vi "get_config_cluster.vi"(8 "error in (no error)":errorcluster, 11 "ScanModeDL090923Scaffold in":refnum<class "ImagingModeDL090923Scaffold.lvclass">) -> (0 "error out":errorcluster, 2 "config cluster (variant)":variant, 3 "ScanModeDL090923Scaffold out":refnum<class "ImagingModeDL090923Scaffold.lvclass">)   [LabVIEW 2010, in "ImagingModeDL090923Scaffold.lvclass"]
uses:
  ImagingModeDL090923Scaffold.lvclass
  ImagingModeDL090923Scaffold.lvclass/ImagingModeDL090923Scaffold.ctl
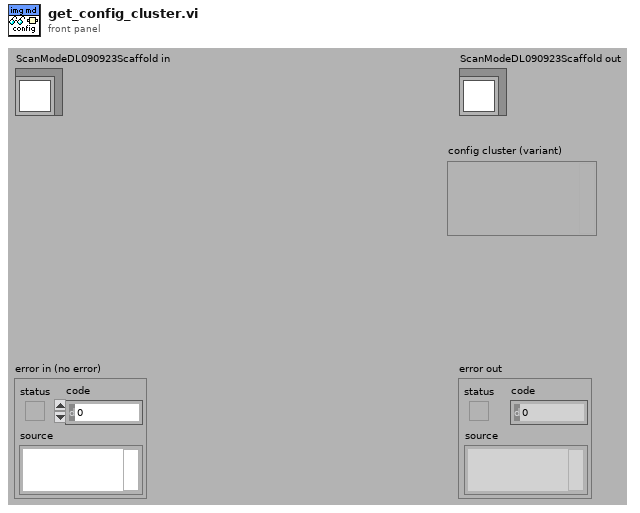
[diagram p1: front panel]
types:
  T1 = typedef "ImagingModeDL090923Scaffold.lvclass/config_data_cluster.ctl" = cluster{"Instrument":T2, "Trajectory":T2, "ScanHead":T2, "DAQ":T2, "ImageAssembler":T2, "DataCollection":T2, "Display":T2, "Analyser":T2, "Stimulator":T2, "Trajectory-to-ImageAssembler adapter path":string, "LSID (cluster)":T4}
  T2 = typedef "ImagingModeDL090923Scaffold.lvclass/component_specification_cluster.ctl" = cluster{"specification":T3, "adapter path":string}
  T3 = typedef "plugin_specification.ctl" = cluster{"class path":string, "configuration":string, "label":string, "settings name":string}
  T4 = typedef "LSID_cluster.ctl" = cluster{"identifier":string, "revision":i32}
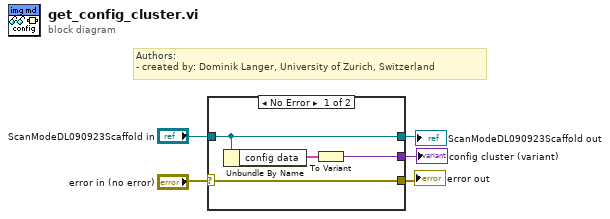
[diagram p0: block diagram]
diagram:
  # "Authors: \n- created by: Dominik Langer, University of Zurich, Switzerland"
  n1 = case shown="No Error" "error in (no error)" {
    selector: "error in (no error)" -> [w8 w10]
    tunnel: "ScanModeDL090923Scaffold in" -> [w9 w11]
    tunnel: [w9 w11] -> w3
    tunnel: [w8 w10] -> w2
    tunnel: [w6 _] -> w1
    frame No Error {
      n2 = Unbundle By Name(w9) -> ("config data"=w7:T1)
      n3 = To Variant(anything=w7) -> (Variant=w6:variant)
    }
    frame Error {
    }
  }
  "error out" <- w2
  "ScanModeDL090923Scaffold out" <- w3
  "config cluster (variant)" <- w1
